vi "Avg2Samps.vi"(4 "channel in":i16[](array[numeric])=[0, 0]) -> (1 "Numeric":i16)   [LabVIEW 2015]
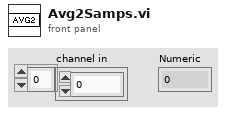
[diagram p1: front panel]
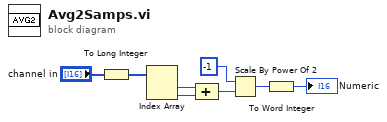
[diagram p0: block diagram]
diagram:
  n1 = To Long Integer(number="channel in") -> (32bit integer=w5:i32[])
  n2 = Index Array(array=w5) -> (element #1=w7:i32, element #2=w6:i32)  [unwired: 2 in]
  n3 = Compound Arithmetic op=ADD(w7, w6) -> (w4:i32)
  n4 = Scale By Power Of 2(n=i16 -1, x=w4) -> (x*2^n=w2:i32)
  n5 = To Word Integer(number=w2) -> (16bit integer=→"Numeric":i16)
